vi "ScpSetTriggerTimeOut.vi"() -> ()   [LabVIEW 2018, in "LibTiePie.lvlib"]
uses:
  LibTiePie.lvlib
  LabViewHS4/libtiepie.dll
panel:
  in  "dTimeOut":dbl
  in  "hDevice":u32
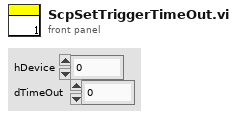
[diagram p1: front panel]
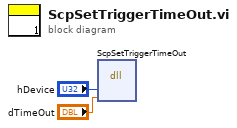
[diagram p0: block diagram]
diagram:
  n1 = dll-call lib="C:/Users/cwaha/Documents/LabViewHS4/libtiepie.dll" fn="ScpSetTriggerTimeOut"("hDevice"="hDevice", "dTimeOut"="dTimeOut") -> ()  [unwired: 6 in, 2 out]
